vi "MessbereichEinstellen.vi"(8 "Error_in":errorcluster, 10 "Channel Name (1: Channel 1)":i32(ring)=1 items=["Channel 1"=1, "Channel 2"=2, "Channel 3"=3, "Channel 4"=4], 11 "VISA Name OZ in(OZ)":refnum<visa-resource-name>="USB0::0x0957::0x179B::MY54313507::INSTR") -> (0 "Error_out":errorcluster, 3 "VISA Name OZ out":refnum<visa-resource-name>)   [LabVIEW 2016]
doc: "Mithilfe dieses VIs wird die Spannung des ausgewählten Channels auf 90% der Größe des Anzeigelements Skaliert. Zudem wird noch der gemessene Sinus auf 2 Perioden skaliert."
panel:
  out "VPP":string
  out "Periodendauer [ms]":dbl
  out "Frequenz_alt":string
  out "Range_final":string
  out "RANGE 2":string
  out "Range_alt":string
  out "VMIN":string
  out "VMAX":string
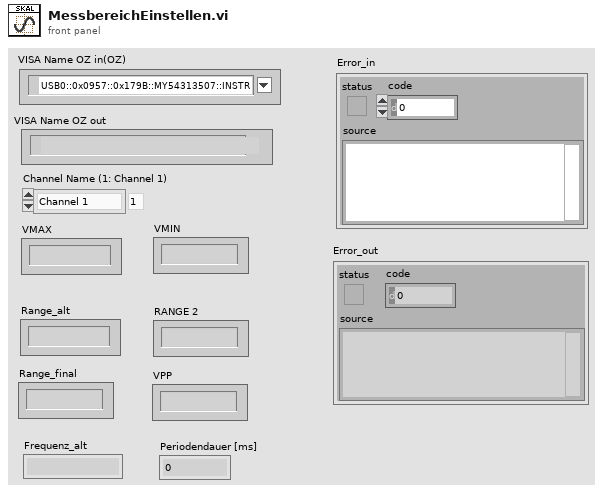
[diagram p1: front panel]
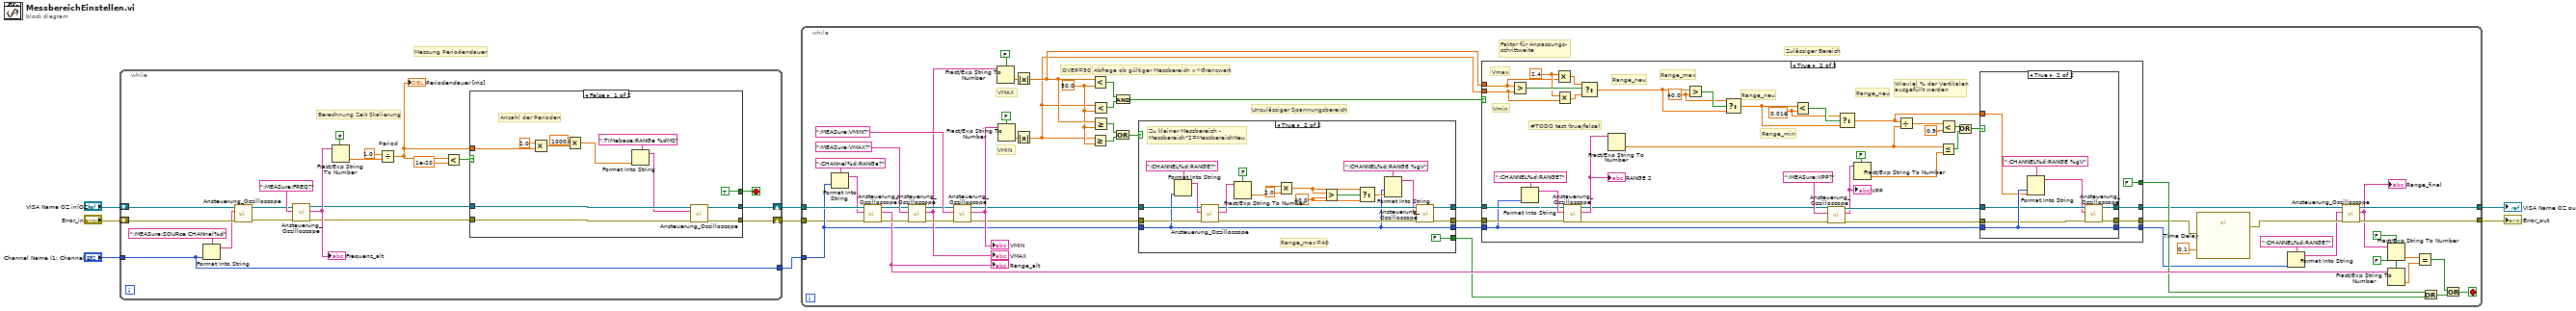
[diagram p0: block diagram]
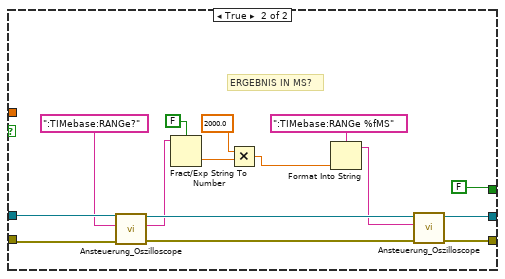
[diagram p2: hidden frame]
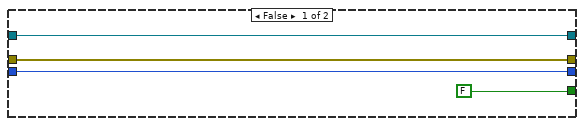
[diagram p3: hidden frame]
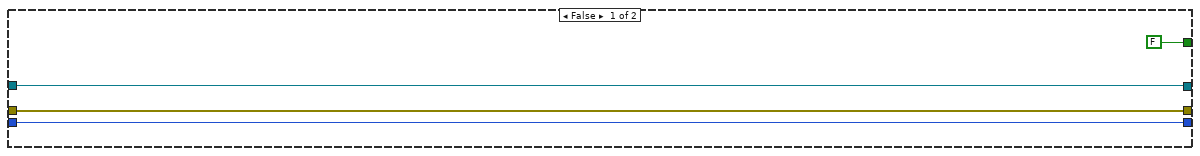
[diagram p4: hidden frame]
diagram:
  # "Messung Periodendauer"
  n1 = while {
    shift-right: [w20] -> w6
    shift-left: "VISA Name OZ in(OZ)" -> [w12]
    shift-right: [w21] -> w2
    shift-left: "Error_in" -> [w13]
    tunnel: "Channel Name (1: Channel 1)" -> [w9]
    tunnel: [w9] -> w1
    stop <- w16 stop-if-true
    # "Berechnung Zeit Skalierung"
    n2 = Format Into String(format string=":MEASure:SOURce CHANnel%d" ("Schreibpuffer"), w9) -> (resulting string=w10:string)  [unwired: 2 in, 1 out]
    n3 = call "Ansteuerung_Oszilloscope.vi"("Error_in"=w13, "Eingangs-String"=w10, "VISA Name OZ in(OZ)"=w12) -> ("Error_out"=w14:errorcluster, "VISA Name OZ out"=w15:refnum<visa-resource-name>)  [unwired: 6 in, 1 out]
    n4 = call "Ansteuerung_Oszilloscope.vi"("Error_in"=w14, "Eingangs-String"=":MEASure:FREQ?" ("Schreibpuffer"), "VISA Name OZ in(OZ)"=w15) -> ("Error_out"=w22:errorcluster, "Ausgangs-String"=w25:string, "VISA Name OZ out"=w23:refnum<visa-resource-name>)  [unwired: 6 in]
    "Frequenz_alt" <- w25
    n5 = Fract/Exp String To Number(use system decimal point (T)=FALSE ("Systemdezimalzeichen verwenden (T)"), string=w25) -> (number=w26:dbl)  [unwired: 2 in, 1 out]
    n6 = Divide "Period"(x=1.0, y=w26) -> (x/y=w18:dbl)
    "Periodendauer [ms]" <- w18
    n7 = Less?(x=w18, y=1e-20) -> (x < y?=w19:bool)
    n8 = case shown="False" w19 {
      tunnel: w18 -> [w35 _]
      tunnel: w23 -> [w34 w50]
      tunnel: w22 -> [w33 w51]
      tunnel: [w32 w52] -> w21
      tunnel: [w31 w53] -> w20
      tunnel: [TRUE FALSE] -> w16
      frame False {
        # "Anzahl der Perioden"
        n9 = Multiply(x=2.0, y=w35) -> (x*y=w38:dbl)
        n10 = Multiply(x=1000.0, y=w38) -> (x*y=w37:dbl)
        n11 = Format Into String(format string=":TIMebase:RANGe %dMS" ("Schreibpuffer"), w37) -> (resulting string=w29:string)  [unwired: 2 in, 1 out]
        n12 = call "Ansteuerung_Oszilloscope.vi"("Error_in"=w33, "Eingangs-String"=w29, "VISA Name OZ in(OZ)"=w34) -> ("Error_out"=w32:errorcluster, "VISA Name OZ out"=w31:refnum<visa-resource-name>)  [unwired: 6 in, 1 out]
      }
      frame True {
        # "ERGEBNIS IN MS?"
        n13 = call "Ansteuerung_Oszilloscope.vi"("Error_in"=w51, "Eingangs-String"=":TIMebase:RANGe?" ("Schreibpuffer"), "VISA Name OZ in(OZ)"=w50) -> ("Error_out"=w54:errorcluster, "Ausgangs-String"=w47:string, "VISA Name OZ out"=w55:refnum<visa-resource-name>)  [unwired: 6 in]
        n14 = Fract/Exp String To Number(use system decimal point (T)=FALSE, string=w47) -> (number=w45:dbl)  [unwired: 2 in, 1 out]
        n15 = Multiply(x=2000.0, y=w45) -> (x*y=w41:dbl)
        n16 = Format Into String(format string=":TIMebase:RANGe %fMS" ("Schreibpuffer"), w41) -> (resulting string=w42:string)  [unwired: 2 in, 1 out]
        n17 = call "Ansteuerung_Oszilloscope.vi"("Error_in"=w54, "Eingangs-String"=w42, "VISA Name OZ in(OZ)"=w55) -> ("Error_out"=w52:errorcluster, "VISA Name OZ out"=w53:refnum<visa-resource-name>)  [unwired: 6 in, 1 out]
      }
    }
  }
  n18 = while {
    tunnel: w6 -> [w90]
    tunnel: [w86] -> w5
    tunnel: [w84] -> w4
    tunnel: w1 -> [w59]
    tunnel: w2 -> [w58]
    stop <- w56 stop-if-true
    w97 = 50.0 ("y")
    # "Faktor für Anpassungs-\nschrittweite"
    # "VMIN"
    # "VMAX"
    # "OVER=50"
    # "Unzulässiger Spannungsbereich"
    # "Zulässiger Bereich"
    # "Abfrage ob gültiger Messbereich x<Grenzwert"
    n19 = Format Into String(format string=":CHANnel%d:RANGe?" ("Schreibpuffer"), w59) -> (resulting string=w88:string)  [unwired: 2 in, 1 out]
    n20 = call "Ansteuerung_Oszilloscope.vi"("Error_in"=w58, "Eingangs-String"=w88, "VISA Name OZ in(OZ)"=w90) -> ("Error_out"=w91:errorcluster, "Ausgangs-String"=w79:string, "VISA Name OZ out"=w92:refnum<visa-resource-name>)  [unwired: 6 in]
    "Range_alt" <- w79
    n21 = call "Ansteuerung_Oszilloscope.vi"("Error_in"=w91, "Eingangs-String"=":MEASure:VMAX?" ("Schreibpuffer"), "VISA Name OZ in(OZ)"=w92) -> ("Error_out"=w106:errorcluster, "Ausgangs-String"=w102:string, "VISA Name OZ out"=w103:refnum<visa-resource-name>)  [unwired: 6 in]
    "VMAX" <- w102
    n22 = call "Ansteuerung_Oszilloscope.vi"("Error_in"=w106, "Eingangs-String"=":MEASure:VMIN?" ("Schreibpuffer"), "VISA Name OZ in(OZ)"=w103) -> ("Error_out"=w66:errorcluster, "Ausgangs-String"=w99:string, "VISA Name OZ out"=w67:refnum<visa-resource-name>)  [unwired: 6 in]
    "VMIN" <- w99
    n23 = Fract/Exp String To Number(use system decimal point (T)=FALSE, string=w102) -> (number=w73:dbl)  [unwired: 2 in, 1 out]
    n24 = Fract/Exp String To Number(use system decimal point (T)=FALSE, string=w99) -> (number=w72:dbl)  [unwired: 2 in, 1 out]
    n25 = Absolute Value(x=w73) -> (abs(x)=w98:dbl)
    n26 = Absolute Value(x=w72) -> (abs(x)=w61:dbl)
    n27 = Less?(x=w98, y=w97) -> (x < y?=w95:bool)
    n28 = Greater Or Equal?(x=w61, y=w97) -> (x >= y?=w93:bool)
    n29 = Less?(x=w61, y=w97) -> (x < y?=w96:bool)
    n30 = Greater Or Equal?(x=w98, y=w97) -> (x >= y?=w94:bool)
    n31 = Or(x=w94, y=w93) -> (x .or. y?=w65:bool)
    n32 = And(x=w95, y=w96) -> (x .and. y?=w71:bool)
    n33 = case shown="True" w65 {
      tunnel: w67 -> [w110 w130]
      tunnel: w66 -> [w109 w122]
      tunnel: w59 -> [w107 w112]
      tunnel: [FALSE FALSE] -> w62
      tunnel: [w109 w115] -> w69
      tunnel: [w110 w114] -> w70
      tunnel: [w107 w112] -> w68
      frame False {
      }
      frame True {
        w117 = 40.0 ("y")
        # "Zu kleiner Messbereich -\nMessbereich*2=MessbereichNeu"
        # "Range_max=40"
        n34 = Format Into String(format string=":CHANNEL%d:RANGE?" ("Schreibpuffer"), w112) -> (resulting string=w120:string)  [unwired: 2 in, 1 out]
        n35 = call "Ansteuerung_Oszilloscope.vi"("Error_in"=w122, "Eingangs-String"=w120, "VISA Name OZ in(OZ)"=w130) -> ("Error_out"=w123:errorcluster, "Ausgangs-String"=w128:string, "VISA Name OZ out"=w124:refnum<visa-resource-name>)  [unwired: 6 in]
        n36 = Fract/Exp String To Number(use system decimal point (T)=FALSE, string=w128) -> (number=w127:dbl)  [unwired: 2 in, 1 out]
        n37 = Multiply(x=w127, y=2.0) -> (x*y=w118:dbl)
        n38 = Greater?(x=w118, y=w117) -> (0:w119:bool)
        n39 = Select(t=w118, s=w119, f=w117) -> (s? t:f=w113:dbl)
        n40 = Format Into String(format string=":CHANNEL%d:RANGE %gV", w112, w113) -> (resulting string=w111:string)  [unwired: 2 in, 1 out]
        n41 = call "Ansteuerung_Oszilloscope.vi"("Error_in"=w123, "Eingangs-String"=w111, "VISA Name OZ in(OZ)"=w124) -> ("Error_out"=w115:errorcluster, "VISA Name OZ out"=w114:refnum<visa-resource-name>)  [unwired: 6 in, 1 out]
      }
    }
    n42 = case shown="True" w71 {
      tunnel: w70 -> [w134 w169]
      tunnel: [w134 w153] -> w64
      tunnel: w69 -> [w133 w168]
      tunnel: [w133 w152] -> w63
      tunnel: [w132 w151] -> w60
      tunnel: w68 -> [w132 w150]
      tunnel: [FALSE FALSE] -> w74
      tunnel: w61 -> [_ w161]
      tunnel: w73 -> [_ w160]
      frame False {
      }
      frame True {
        w155 = 0.016 ("y")
        w157 = 40.0 ("y")
        w162 = 2.4 ("y")
        # "Wieviel % der Vertikalen\nausgefüllt werden"
        # "Vmin"
        # "Vmax"
        # "#TODO test (true/false)"
        # "Range_neu"
        # "Range_min"
        # "Range_neu"
        # "Range_max"
        # "Range_neu"
        n43 = Greater?(x=w160, y=w161) -> (0:w165:bool)
        n44 = Format Into String(format string=":CHANNEL%d:RANGE?" ("Schreibpuffer"), w150) -> (resulting string=w170:string)  [unwired: 2 in, 1 out]
        n45 = Multiply(x=w162, y=w160) -> (x*y=w164:dbl)
        n46 = Multiply(x=w162, y=w161) -> (x*y=w163:dbl)
        n47 = call "Ansteuerung_Oszilloscope.vi"("Error_in"=w168, "Eingangs-String"=w170, "VISA Name OZ in(OZ)"=w169) -> ("Error_out"=w141:errorcluster, "Ausgangs-String"=w167:string, "VISA Name OZ out"=w144:refnum<visa-resource-name>)  [unwired: 6 in]
        "RANGE 2" <- w167
        n48 = Select(t=w164, s=w165, f=w163) -> (s? t:f=w158:dbl)
        n49 = Fract/Exp String To Number(string=w167) -> (number=w135:dbl)  [unwired: 3 in, 1 out]
        n50 = Greater?(x=w158, y=w157) -> (0:w159:bool)
        n51 = Select(t=w157, s=w159, f=w158) -> (s? t:f=w154:dbl)
        n52 = Less?(x=w154, y=w155) -> (x < y?=w156:bool)
        n53 = call "Ansteuerung_Oszilloscope.vi"("Error_in"=w141, "Eingangs-String"=":MEASure:VPP?" ("Schreibpuffer"), "VISA Name OZ in(OZ)"=w144) -> ("Error_out"=w142:errorcluster, "Ausgangs-String"=w137:string, "VISA Name OZ out"=w143:refnum<visa-resource-name>)  [unwired: 6 in]
        "VPP" <- w137
        n54 = Select(t=w155, s=w156, f=w154) -> (s? t:f=w148:dbl)
        n55 = Fract/Exp String To Number(use system decimal point (T)=FALSE, string=w137) -> (number=w139:dbl)  [unwired: 2 in, 1 out]
        n56 = Divide(x=w148, y=w135) -> (x/y=w149:dbl)
        n57 = Less Or Equal?(x=w135, y=w139) -> (x <= y?=w138:bool)
        n58 = Less?(x=w149, y=0.9) -> (x < y?=w146:bool)
        n59 = Or(x=w146, y=w138) -> (x .or. y?=w147:bool)
        n60 = case shown="True" w147 {
          tunnel: [w174 w181] -> w153
          tunnel: [w173 w180] -> w152
          tunnel: [w172 w179] -> w151
          tunnel: w150 -> [w172 w179]
          tunnel: w143 -> [w174 w178]
          tunnel: w142 -> [w173 w177]
          tunnel: w148 -> [_ w176]
          frame False {
          }
          frame True {
            n61 = Format Into String(format string=":CHANNEL%d:RANGE %gV" ("Schreibpuffer"), w179, w176) -> (resulting string=w175:string)  [unwired: 2 in, 1 out]
            n62 = call "Ansteuerung_Oszilloscope.vi"("Error_in"=w177, "Eingangs-String"=w175, "VISA Name OZ in(OZ)"=w178) -> ("Error_out"=w180:errorcluster, "VISA Name OZ out"=w181:refnum<visa-resource-name>)  [unwired: 6 in, 1 out]
          }
        }
      }
    }
    n63 = call "Time Delay"("error in (no error)"=w63, "Delay Time (s)"=0.1) -> ("error out"=w85:errorcluster)  [unwired: 9 in]
    n64 = Format Into String(format string=":CHANNEL%d:RANGE?" ("Schreibpuffer"), w60) -> (resulting string=w82:string)  [unwired: 2 in, 1 out]
    n65 = call "Ansteuerung_Oszilloscope.vi"("Error_in"=w85, "Eingangs-String"=w82, "VISA Name OZ in(OZ)"=w64) -> ("Error_out"=w84:errorcluster, "Ausgangs-String"=w57:string, "VISA Name OZ out"=w86:refnum<visa-resource-name>)  [unwired: 6 in]
    "Range_final" <- w57
    n66 = Fract/Exp String To Number(use system decimal point (T)=FALSE, string=w57) -> (number=w78:dbl)  [unwired: 2 in, 1 out]
    n67 = Fract/Exp String To Number(use system decimal point (T)=FALSE, string=w79) -> (number=w77:dbl)  [unwired: 2 in, 1 out]
    n68 = Equal?(x=w78, y=w77) -> (x = y?=w75:bool)
    n69 = Or(x=w74, y=w62) -> (x .or. y?=w76:bool)
    n70 = Or(x=w75, y=w76) -> (x .or. y?=w56:bool)
  }
  "VISA Name OZ out" <- w5
  "Error_out" <- w4
